vi "turn_back.vi"(5 "Motors 2":T1=-1, 7 "Motors":T1=-1, 9 "NXT/EV3":T3, 10 "Gyro Port":T2 items=["Port 1", "Port 2", "Port 3", "Port 4"]) -> (0 "x = y?":bool)   [LabVIEW 2016]
uses:
  <vilib>/NXT/Subs/LVHSConnector.ctl
  <vilib>/NXT/LegoClasses/BrickReference/BrickReference.lvclass
  <vilib>/NXT/Block Support/NXT_InputPort.ctl
  <vilib>/NXT/Hardware/Plugins/Open Port/OpenPortAddress.ctl
  <vilib>/NXT/Block Support/NXT_OutputPort.ctl
  <vilib>/NXT/Dual Mode Library/Sensors/EV3_Gyro_Reset.vi
  <vilib>/NXT/Dual Mode Library/Sensors/EV3_Gyro_Angle.vi
  <vilib>/NXT/NXTIO Xnodes/NXTIONodeSubVIs/NXTMoveMotors.vi
  <vilib>/NXT/NXTIO Xnodes/AddressXNode/NXTIOAddress.xnode
  <vilib>/NXT/NXTIO Xnodes/NXTIOXNode/NXTIO.xnode
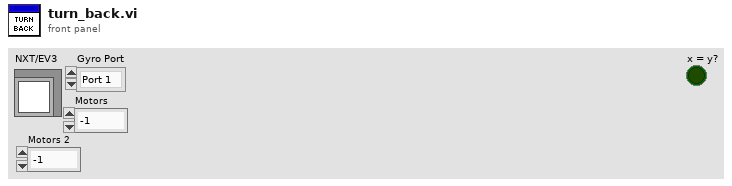
[diagram p1: front panel]
types:
  T1 = typedef "OpenPortAddress.ctl" = i32
  T2 = typedef "NXT_InputPort.ctl" = u32
  T3 = typedef "LVHSConnector.ctl" = refnum<class "BrickReference.lvclass">
  T4 = typedef "NXT_OutputPort.ctl" = u8
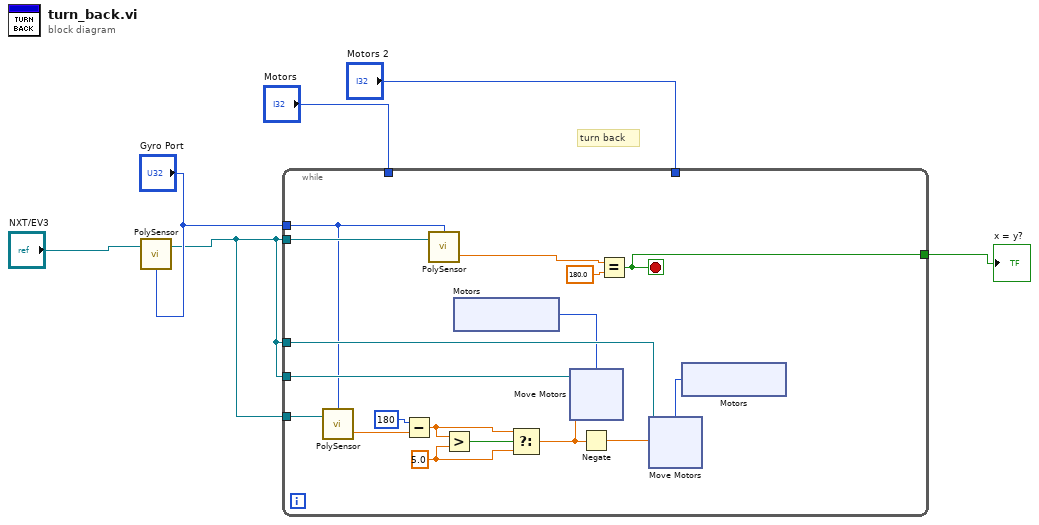
[diagram p0: block diagram]
diagram:
  # "turn back"
  n1 = call-poly <vilib>:"PolySensor.vi"("NXT/EV3"="NXT/EV3", "Port (Port 1)"="Gyro Port") -> ("NXT/EV3"=w1:T3)  [unwired: 2 in]
  n2 = while {
    tunnel: w1 -> [w14]
    tunnel: w1 -> [w13]
    tunnel: w1 -> [w12]
    tunnel: "Gyro Port" -> [w11]
    tunnel: "Motors" -> [_]
    tunnel: "Motors 2" -> [_]
    tunnel: w1 -> [w10]
    tunnel: [w9] -> w4
    stop <- w9 stop-if-true
    w16 = sgl 5.0 ("y")
    n3 = call-poly <vilib>:"PolySensor.vi"("NXT/EV3"=w10, "Port (Port 1)"=w11) -> ("Degrees"=w19:sgl)  [unwired: 1 in, 1 out]
    n4 = Subtract(x=180, y=w19) -> (x-y=w17:sgl)
    n5 = call-poly <vilib>:"PolySensor.vi"("NXT/EV3"=w14, "Port (Port 1)"=w11) -> ("Degrees"=w23:sgl)  [unwired: 1 in, 1 out]
    n6 = Greater?(x=w17, y=w16) -> (0:w18:bool)
    n7 = xnode "Motors"() -> ("Motor"=w8:T4)
    n8 = Select(t=w17, s=w18, f=w16) -> (s? t:f=w15:sgl)
    n9 = xnode "Move Motors"("Power/Speed 1"=w15, "Motors"=w8, "NXT/EV3"=w13) -> ()  [unwired: 1 out]
    n10 = Negate(x=w15) -> (-x=w21:sgl)
    n11 = Equal?(x=w23, y=sgl 180.0) -> (x = y?=w9:bool)
    n12 = xnode "Motors"() -> ("Motor"=w7:T4)
    n13 = xnode "Move Motors"("Power/Speed 1"=w21, "Motors"=w7, "NXT/EV3"=w12) -> ()  [unwired: 1 out]
  }
  "x = y?" <- w4
